vi "K_C_F_units_changer.vi"(10 "temp in":dbl, 11 "Select [°C/°F/K]":enum16{"Celcius", "Farenheit", "Kelvin"}(ring)) -> (3 "temp out":dbl)   [LabVIEW 2024]
uses:
  <vilib>/express/express arith-compare/Formula/XNode/ExpressFormulaBlockNode.xnode
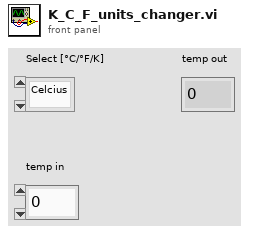
[diagram p1: front panel]
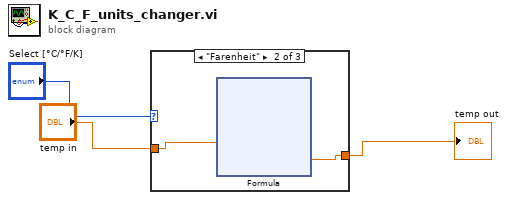
[diagram p0: block diagram]
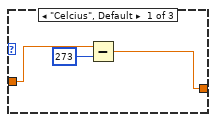
[diagram p2: hidden frame]
diagram:
  n1 = case shown="\"Farenheit\"" "Select [°C/°F/K]" {
    tunnel: [w4 w7 w17] -> w3
    tunnel: "temp in" -> [w6 w8 w17]
    frame "Celcius", Default {
      n2 = Subtract(x=w6, y=273) -> (x-y=w4:dbl)
    }
    frame "Farenheit" {
      n3 = xnode "Formula"("X1"=w8) -> ("Result"=w7:dbl)  [unwired: 1 in, 1 out]
    }
    frame "Kelvin" {
    }
  }
  "temp out" <- w3
